vi "IMAQ Example.vi"() -> ()   [LabVIEW 2020]
uses:
  g_industrial_cam/Camera/Camera.lvclass/Camera.ctl
  g_industrial_cam/Buffer/Buffer.lvclass/Buffer.ctl
  g_industrial_cam/Buffer Byte-Stream Access/Buffer Byte-Stream Access.lvclass/Buffer Byte-Stream Access.ctl
  g_industrial_cam/Buffer/Read Data as Mono10 Image.vi
  g_industrial_cam/Buffer/Read Data as Mono8 Image.vi
  g_industrial_cam/Camera/GetSetPixelFormat.vi
  g_industrial_cam/Buffer/Create from Handle.vi
  g_industrial_cam/Buffer/Access Handle.vi
  g_industrial_cam/Buffer/ReadDataAsMono2Byte.vi
  g_industrial_cam/Camera/Check Not Disconnected.vi
  <vilib>/Utility/error.llb/Error Cluster From Error Code.vi
  g_industrial_cam/Buffer/Buffer.lvclass
  g_industrial_cam/Buffer Byte-Stream Access/Buffer Byte-Stream Access.lvclass
  g_industrial_cam/Camera/Camera.lvclass
panel:
  in  "Bit Depth":enum16{"Mono10", "Mono8"}(ring)
  out "Copy Array":T1(plugin-control)
  out "Byte Stream":T1(plugin-control)
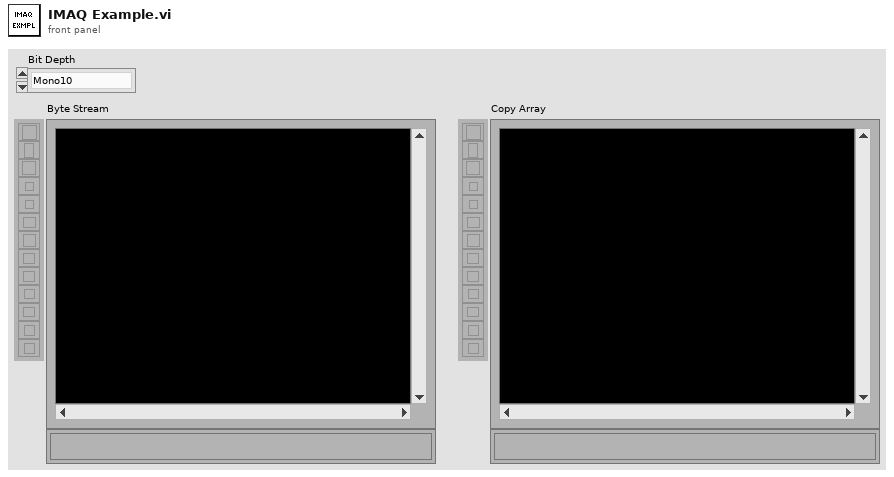
[diagram p1: front panel]
types:
  T1 = typedef "IMAQ Image.ctl" = refnum<image>
  T2 = typedef "Device Enumeration.ctl" = cluster{"ID":string, "Protocol":string, "Vendor":string, "Model":string, "Serial":string, "Address":string}
  T3 = typedef "Image Type" = u32
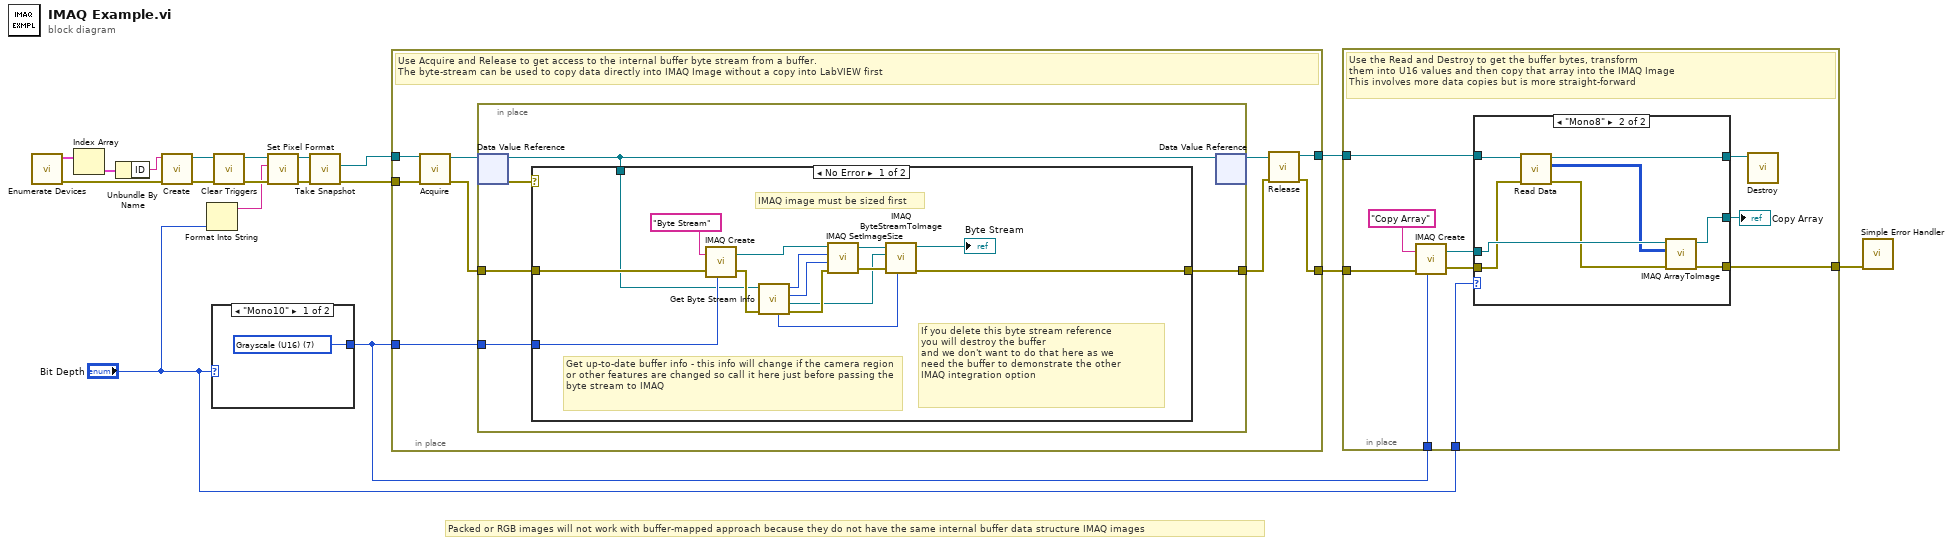
[diagram p0: block diagram]
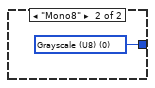
[diagram p2: hidden frame]
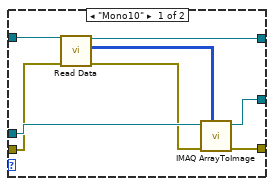
[diagram p4: hidden frame]
diagram:
  # "Packed or RGB images will not work with buffer-mapped approach because they do not have the same internal buffer data structure IMAQ images"
  n1 = call "Enumerate Devices.vi"() -> ("error out"=w16:errorcluster, "Devices"=w18:T2[])  [unwired: 10 in]
  n2 = Index Array(array=w18) -> (element=w17:T2)  [unwired: 1 in]
  n3 = Unbundle By Name(w17) -> ("ID"=w15:string)
  n4 = call "Create.vi"("error in (no error)"=w16, "Identifier (ID, IP etc)"=w15) -> ("error out"=w14:errorcluster, "Camera"=w13:refnum<class "Camera.lvclass">)  [unwired: 8 in]
  n5 = Format Into String("Bit Depth") -> (resulting string=w4:string)  [unwired: 3 in, 1 out]
  n6 = case shown="\"Mono10\"" "Bit Depth" {
    tunnel: [w19 w20] -> w3
    frame "Mono10" {
      w19 = T3 7 items=["Grayscale (U8)", "Grayscale (I16)", "Grayscale (SGL)", "Complex (CSG)", "RGB (U32)", "HSL (U32)", "RGB (U64)", "Grayscale (U16)"] ("Image Type")
    }
    frame "Mono8" {
      w20 = T3 0 items=["Grayscale (U8)", "Grayscale (I16)", "Grayscale (SGL)", "Complex (CSG)", "RGB (U32)", "HSL (U32)", "RGB (U64)", "Grayscale (U16)"] ("Image Type")
    }
  }
  n7 = call "Clear Triggers.vi"("error in (no error)"=w14, "Camera in"=w13) -> ("error out"=w12:errorcluster, "Camera"=w11:refnum<class "Camera.lvclass">)  [unwired: 8 in]
  n8 = call "Set Pixel Format.vi"("error in (no error)"=w12, "Pixel Format"=w4, "Camera in"=w11) -> ("error out"=w10:errorcluster, "Camera"=w9:refnum<class "Camera.lvclass">)  [unwired: 7 in]
  n9 = call "Take Snapshot.vi"("error in (no error)"=w10, "Camera in"=w9) -> ("error out"=w7:errorcluster, "New Buffer"=w8:refnum<class "Buffer.lvclass">)  [unwired: 7 in, 1 out]
  n10 = in-place {
    in-place-border: [w22] -> w6
    in-place-border: w8 -> [w28]
    in-place-border: w7 -> [w29]
    in-place-border: w3 -> [w27]
    in-place-border: [w21] -> w1
    # "Use Acquire and Release to get access to the internal buffer byte stream from a buffer.\nThe byte-stream can be used to copy data directly into IMAQ Image without a copy into LabVIEW first"
    n11 = call "Acquire.vi"("error in (no error)"=w29, "Buffer in"=w28) -> ("error out"=w25:errorcluster, "Mapped Buffer"=w26:refnum<data-value>)  [unwired: 8 in]
    n12 = in-place {
      in-place-border: [w34] -> w23
      in-place-border: w27 -> [w33]
      in-place-border: w25 -> [w31]
      n13 = in-place-dvr #1(w26) -> (w30:refnum<class "Buffer Byte-Stream Access.lvclass">, w32:errorcluster)
      n14 = case shown="No Error" w32 {
        selector: w32 -> [_ w50]
        tunnel: [w43 w50] -> w34
        tunnel: w33 -> [w41 _]
        tunnel: w31 -> [w40 _]
        tunnel: w30 -> [w39 _]
        frame No Error {
          # "If you delete this byte stream reference\nyou will destroy the buffer\nand we don't want to do that here as we\nneed the buffer to demonstrate the other\nIMAQ integration option"
          # "Get up-to-date buffer info - this info will change if the camera region or other features are changed so call it here just before passing the byte stream to IMAQ"
          # "IMAQ image must be sized first"
          n15 = call "IMAQ Create"("Image Name"="Byte Stream", "Image Type"=w41, "error in (no error)"=w40) -> ("New Image"=w45:T1, "error out"=w48:errorcluster)  [unwired: 2 in]
          n16 = call "Get Byte Stream Info.vi"("error in (no error)"=w48, "Mapped-Buffer"=w39) -> ("error out"=w49:errorcluster, "Byte Stream (Do Not Delete)"=w36:refnum<data-value>, "Y Resolution"=w37:i32, "X Resolution"=w38:i32, "Bytes to Copy"=w35:u64)  [unwired: 5 in]
          n17 = call "IMAQ SetImageSize"("error in (no error)"=w49, "Y Resolution"=w37, "X Resolution"=w38, "Image"=w45) -> ("error out"=w47:errorcluster, "Image Out"=w44:T1)  [unwired: 1 in]
          n18 = call "IMAQ ByteStreamToImage"("Bytes to Copy"=w35, "error in (no error)"=w47, "Byte Stream In"=w36, "Image In"=w44) -> ("error out"=w43:errorcluster, "Image Out"=→"Byte Stream":T1)  [unwired: 3 in, 3 out]
        }
        frame Error {
        }
      }
      n19 = in-place-dvr #1(w30) -> (w24:refnum<data-value>)  [unwired: 1 out]
    }
    n20 = call "Release.vi"("error in (no error)"=w23, "Mapped Buffer"=w24) -> ("error out"=w22:errorcluster, "Buffer"=w21:refnum<class "Buffer.lvclass">)  [unwired: 8 in]
  }
  n21 = in-place {
    in-place-border: w6 -> [w53]
    in-place-border: [w56] -> w5
    in-place-border: w3 -> [w55]
    in-place-border: "Bit Depth" -> [w54]
    in-place-border: w1 -> [w51]
    # "Use the Read and Destroy to get the buffer bytes, transform\nthem into U16 values and then copy that array into the IMAQ Image\nThis involves more data copies but is more straight-forward"
    n22 = call "IMAQ Create"("Image Name"="Copy Array", "Image Type"=w55, "error in (no error)"=w53) -> ("New Image"=w59:T1, "error out"=w58:errorcluster)  [unwired: 2 in]
    n23 = case shown="\"Mono8\"" w54 {
      tunnel: w59 -> [w68 w76]
      tunnel: w58 -> [w65 w73]
      tunnel: [w67 w75] -> w57
      tunnel: [w66 w74] -> w56
      tunnel: [w62 w70] -> w52
      tunnel: w51 -> [w61 w69]
      frame "Mono10" {
        n24 = call-poly "Read Data.vi"("error in (no error)"=w65, "Buffer in"=w61) -> ("error out"=w64:errorcluster, "Image"=w63:u16[][], "Buffer"=w62:refnum<class "Buffer.lvclass">)  [unwired: 7 in]
        n25 = call "IMAQ ArrayToImage"("Image Pixels (U16)"=w63, "error in (no error)"=w64, "Image"=w68) -> ("error out"=w66:errorcluster, "Image Out"=w67:T1)  [unwired: 7 in]
      }
      frame "Mono8" {
        n26 = call-poly "Read Data.vi"("error in (no error)"=w73, "Buffer in"=w69) -> ("error out"=w72:errorcluster, "Image"=w71:u8[][], "Buffer"=w70:refnum<class "Buffer.lvclass">)  [unwired: 7 in]
        n27 = call "IMAQ ArrayToImage"("error in (no error)"=w72, "Image Pixels (U8)"=w71, "Image"=w76) -> ("error out"=w74:errorcluster, "Image Out"=w75:T1)  [unwired: 7 in]
      }
    }
    "Copy Array" <- w57
    n28 = call "Destroy.vi"("Buffer in"=w52) -> ()  [unwired: 10 in, 1 out]
  }
  n29 = call <vilib>:"Simple Error Handler.vi"("error in (no error)"=w5) -> ()  [unwired: 4 in, 5 out]
